vi "myRIO v1.0 Scaling Constants Table.vi"() -> ()   [LabVIEW 2021]
panel:
  in  "myRIO 1.0 Scaling Constant Table":string="Not Connected;0;0;0\nA/AI0;1220703;0;0\nA/AI1;1220703;0;0\nA/AI2;1220703;0;0\nA/AI3;1220703;0;0\nB/AI0;1220703;0;0\nB/AI1;1220703;0;0\nB/AI2;1220703;0;0\nB/AI3;1220703;0;0\nC/AI0;4882813;0;1\nC/AI1;4882813;0;1\nAudioIn/Left;1220703;0;1\nAudioIn/Right;1220703;0;1\nA/AO0;1220703;0;0\nA/AO1;1220703;0;0\nB/AO0;1220703;0;0\nB/AO1;1220703;0;0\nC/AO0;4882813;0;1\nC/AO1;4882813;0;1\nAudioOut/Left;1220703;0;1\nAudioOut/Right;1220703;0;1\nONBOARD/ACC;256\nA/AI0 (N Samples);1220703;0;0\nAudioIn/Left (N Samples);1220703;0;1\nAudioIn/Right (N Samples);1220703;0;1\nA/AO0 (N Samples);1220703;0;0\nAudioOut/Left (N Samples);1220703;0;1\nAudioOut/Right (N Samples);1220703;0;1\nA/AI0 (Interrupt);1220703;0;0\nA/AI1 (Interrupt);1220703;0;0"
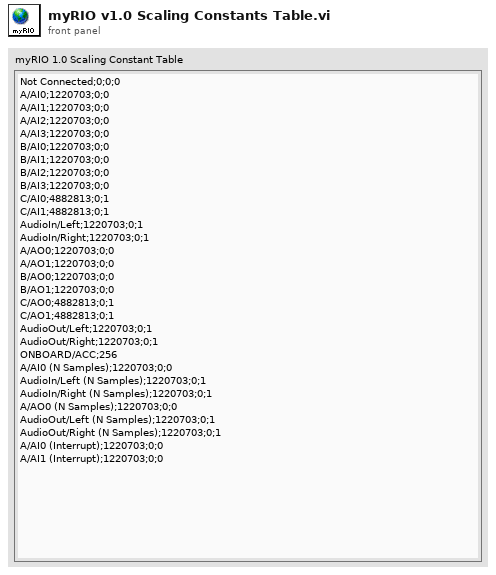
[diagram p1: front panel]
diagram:
